vi "WSVCAP SHL Host LL Manage FPGA Top Level Controls Instantiated Wrapper.vi"(0 "Value In":variant, 1 "FPGA VI Reference (Init Only)":T2, 7 "FPGA Top Level Control":T3=enum."Read Status Flag", 11 "error in (no error)":errorcluster, 12 "Simulate FPGA (Init Only)":bool=TRUE, 13 "Operation":T4, 14 "FPGA":T1) -> (4 "Value Out":variant, 15 "error out":errorcluster)   [LabVIEW 2012]
uses:
  Type Defs/WSVCAP SHL Top Level Control Operation Enum.ctl
  Type Defs/WSVCAP SHL Top Level Control Enum.ctl
  Type Defs/WSVCAP SHL FPGA VI Reference.ctl
  Type Defs/WSVCAP SHL I2C FPGA Enum.ctl
  user.lib/Utilities/Type Defs/MISC Instance Manager Operation.ctl
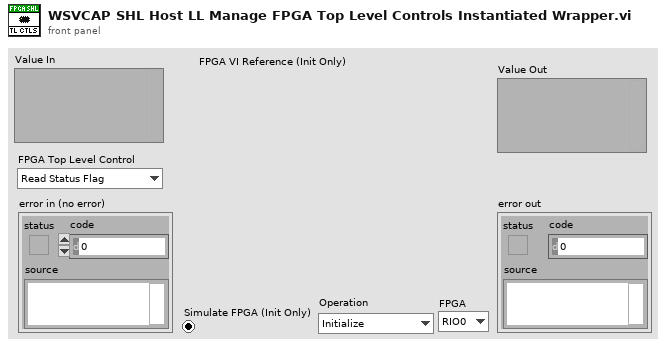
[diagram p1: front panel]
types:
  T1 = typedef "WSVCAP SHL I2C FPGA Enum.ctl" = enum16{"RIO0", "RIO1"}
  T2 = typedef "WSVCAP SHL FPGA VI Reference.ctl" = refnum<k20>
  T3 = typedef "WSVCAP SHL Top Level Control Enum.ctl" = enum16{"Start", "Cmd", "Transaction", "Wait Ticks", "Socket Mask", "UUT Set", "Slave Address", "Sub Address", "Bytes to Write", "Bytes to Read", "Write Data", "Write Flag", "Read Data", "Read Flag", "Ack Read", "Read Status Flag", "Ack Read Status", "Status", "Cycle Count", "Stop Cycle", "Exit"}
  T4 = typedef "WSVCAP SHL Top Level Control Operation Enum.ctl" = enum16{"Initialize", "Set Control", "Read Control", "Close"}
  T5 = typedef "MISC Instance Manager Operation.ctl" = enum16{"Create Instance", "Get Instance ID"}
  T6 = typedef "WSVCAP SHL Manage FPGA Top Level Controls VI Ref.ctl" = refnum<vi>
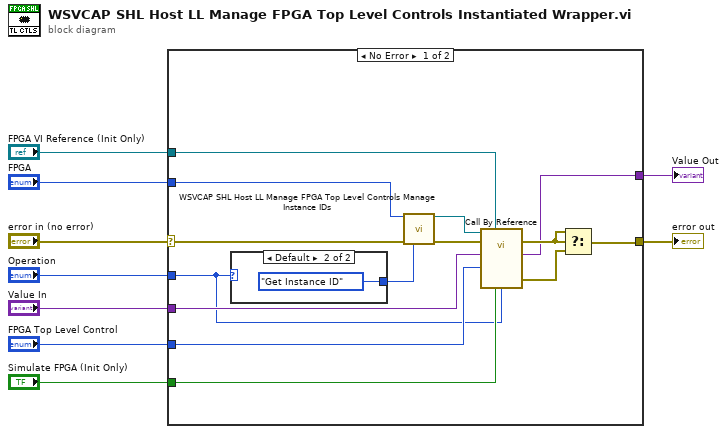
[diagram p0: block diagram]
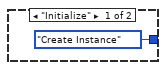
[diagram p2: hidden frame]
diagram:
  n1 = case shown="No Error" "error in (no error)" {
    selector: "error in (no error)" -> [w21 w26]
    tunnel: [w17 w26] -> w1
    tunnel: "Operation" -> [w10 _]
    tunnel: "FPGA" -> [w16 _]
    tunnel: "FPGA VI Reference (Init Only)" -> [w15 _]
    tunnel: "Value In" -> [w14 _]
    tunnel: "Simulate FPGA (Init Only)" -> [w13 _]
    tunnel: "FPGA Top Level Control" -> [w12 _]
    tunnel: [w11 _] -> w2
    frame No Error {
      n2 = case shown="Default" w10 {
        tunnel: [MISC_Instance_Manager_Operation."Create Instance" ("Operation") MISC_Instance_Manager_Operation."Get Instance ID" ("Operation")] -> w19
        frame "Initialize" {
        }
        frame Default {
        }
      }
      n3 = call "WSVCAP SHL Host LL Manage FPGA Top Level Controls Manage Instance IDs.vi"("FPGA"=w16, "error in (no error)"=w21, "Operation"=w19) -> ("VI Ref"=w18:T6, "error out"=w20:errorcluster)  [unwired: 11 in]
      n4 = call-by-ref "?"(reference=w18, error in=w20, "Value In"=w14, "FPGA VI Reference (Init Only)"=w15, "FPGA Top Level Control"=w12, "Simulate FPGA (Init Only)"=w13, "Operation"=w10) -> (error out=w22:errorcluster, "Value Out"=w11:variant, 15:"error out"=w23:errorcluster)  [unwired: 9 in, 1 out]
      n5 = Select(t=w22, s=w22, f=w23) -> (s? t:f=w17:errorcluster)
    }
    frame Error {
    }
  }
  "error out" <- w1
  "Value Out" <- w2
